vi "Initialize.vi"(0 "VISA resource name":refnum<visa-resource-name>, 1 "ID Query (True)":bool=TRUE, 2 "Reset (False)":bool, 3 "error in (no error)":errorcluster, 4 "Serial Link (RS232)":enum16{"RS232", "USB"}(ring)) -> (7 "VISA resource name out":refnum<visa-resource-name>, 8 "Cleared Error Queue":string, 10 "error out":errorcluster {"code" format="%.0x"})   [LabVIEW 2011, in "Newport ESP301.lvlib"]
doc: "Establishes communication with the instrument and optionally performs an instrument identification query and/or an instrument reset. It also places the instrument in a default state needed for other instrument driver operations. Therefore, call this VI before calling other instrument driver VIs for this instrument. Generally, you need to call the Initialize VI only once at the beginning of an application."
uses:
  Newport ESP301.lvlib
panel:
  # "(c) 2009 <Newport>.  ALL RIGHTS RESERVED."
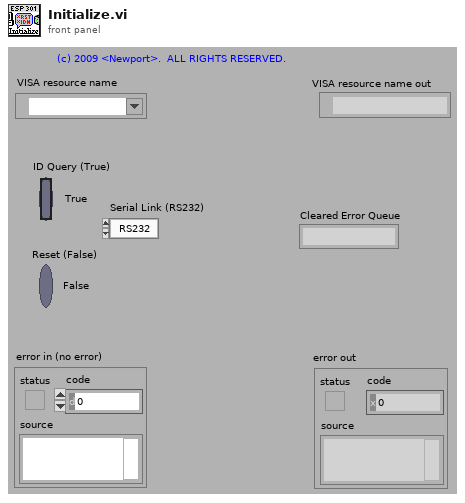
[diagram p1: front panel]
types:
  T1 = cluster{"Baud Rate":u32, "Parity":u16, "Data Bits":u16, "Stop Bits":u16, "Flow Control":u16}
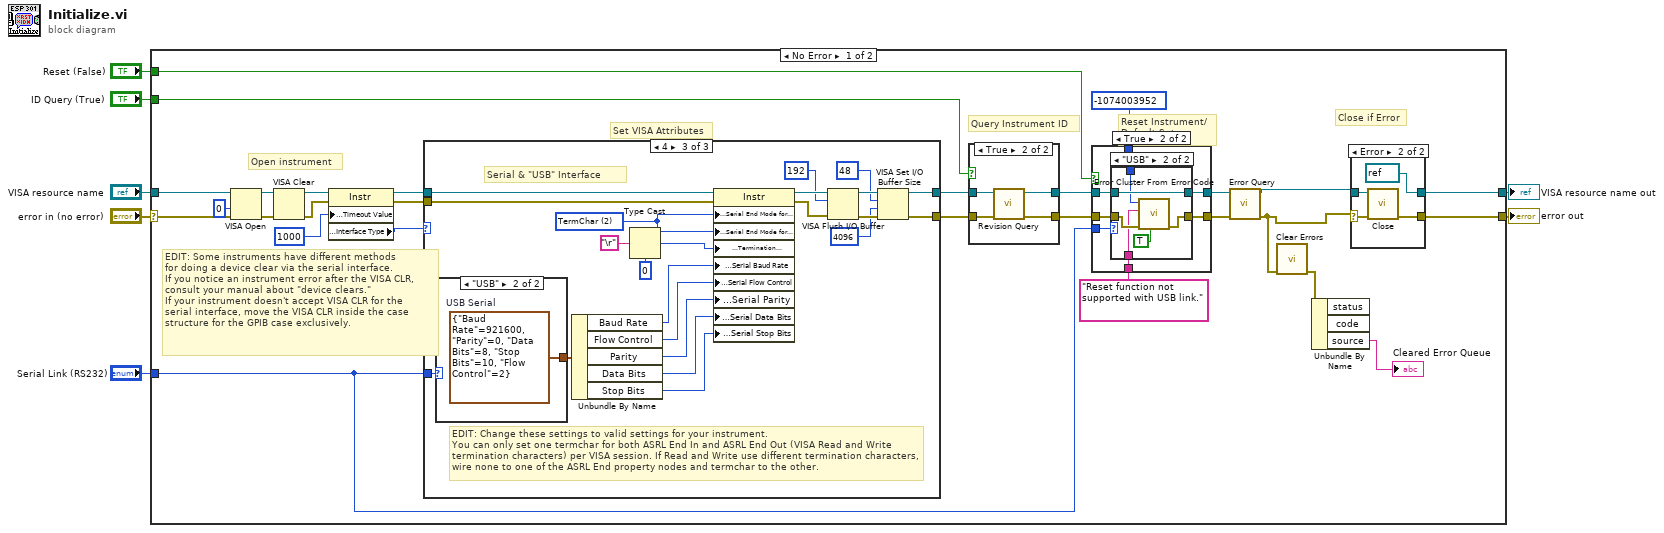
[diagram p0: block diagram]
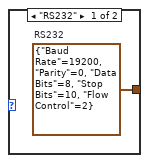
[diagram p5: hidden frame]
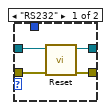
[diagram p7: hidden frame]
diagram:
  n1 = case shown="No Error" "error in (no error)" {
    selector: "error in (no error)" -> [w17 w96]
    tunnel: "ID Query (True)" -> [w33 _]
    tunnel: "Reset (False)" -> [w32 _]
    tunnel: "VISA resource name" -> [w31 w95]
    tunnel: [w15 w95] -> w4
    tunnel: [w16 w96] -> w3
    tunnel: "Serial Link (RS232)" -> [w14 _]
    frame No Error {
      # "EDIT: Some instruments have different methods\nfor doing a device clear via the serial interface.  \nIf you notice an instrument error after the VISA CLR,\nconsult your manual about \"device clears.\"  \nIf your instrument doesn't accept VISA CLR for the\nserial interface, move the VISA CLR inside the case \nstructure for the GPIB case exclusively."
      # "Set VISA Attributes"
      # "Close if Error"
      # "Query Instrument ID"
      # "Reset Instrument/\nDefault Setup"
      # "Open instrument"
      n2 = VISA Open(access mode=u32 0, error in (no error)=w17, VISA resource name=w31) -> (VISA resource name=w24:refnum<visa-resource-name>, error out=w23:errorcluster)  [unwired: 2 out]
      n3 = VISA Clear(VISA resource name=w24, error in (no error)=w23) -> (VISA resource name out=w22:refnum<visa-resource-name>, error out=w21:errorcluster)
      n4 = property class="Instr"(reference=w22, error in=w21, "General Settings:Timeout Value"=u32 1000) -> (reference out=w27:refnum<visa-resource-name>, error out=w26:errorcluster, "Interface Information:Interface Type"=w18:u16)
      n5 = case shown="4" w18 {
        tunnel: [w42 w45 w64] -> w29
        tunnel: [w43 w44 w61] -> w28
        tunnel: w27 -> [w42 w45 w66]
        tunnel: w26 -> [w43 w44 w67]
        tunnel: w14 -> [_ _ w48]
        frame Default {
          # "TCP/IP, and USB Interface"
        }
        frame 1 {
          # "GPIB Interface"
        }
        frame 4 {
          w55 = u16 2 items=["None", "LastBit", "TermChar"] ("Serial Settings:Serial End Mode for Reads")
          # "EDIT: Change these settings to valid settings for your instrument.\nYou can only set one termchar for both ASRL End In and ASRL End Out (VISA Read and Write termination characters) per VISA session. If Read and Write use different termination characters, wire none to one of the ASRL End property nodes and termchar to the other."
          # "Serial & \"USB\" Interface"
          n6 = case shown="\"USB\"" w48 {
            tunnel: [w68 w69] -> w47
            frame "RS232" {
              w68 = T1 {"Baud Rate"=19200, "Parity"=0, "Data Bits"=8, "Stop Bits"=10, "Flow Control"=2}  # RS232
            }
            frame "USB" {
              w69 = T1 {"Baud Rate"=921600, "Parity"=0, "Data Bits"=8, "Stop Bits"=10, "Flow Control"=2}  # USB Serial
            }
          }
          n7 = Unbundle By Name(w47) -> ("Baud Rate"=w53:u32, "Flow Control"=w50:u16, "Parity"=w51:u16, "Data Bits"=w52:u16, "Stop Bits"=w49:u16)
          n8 = Type Cast(type=u8 0, x="\r") -> (*(type *) &x=w54:u8)
          n9 = property class="Instr"(reference=w66, error in=w67, "Serial Settings:Serial End Mode for Reads"=w55, "Serial Settings:Serial End Mode for Writes"=w55, "Message Based Settings:Termination Character"=w54, "Serial Settings:Serial Baud Rate"=w53, "Serial Settings:Serial Flow Control"=w50, "Serial Settings:Serial Parity"=w51, "Serial Settings:Serial Data Bits"=w52, "Serial Settings:Serial Stop Bits"=w49) -> (reference out=w60:refnum<visa-resource-name>, error out=w63:errorcluster)
          n10 = VISA Flush I/O Buffer(VISA resource name=w60, mask (16)=u16 192, error in (no error)=w63) -> (VISA resource name out=w65:refnum<visa-resource-name>, error out=w62:errorcluster)
          n11 = VISA Set I/O Buffer Size(VISA resource name=w65, mask (16)=u16 48, size (4096)=u32 4096 ("size (0)"), error in (no error)=w62) -> (VISA resource name out=w64:refnum<visa-resource-name>, error out=w61:errorcluster)
        }
      }
      n12 = case shown="True" w33 {
        tunnel: [w89 w91] -> w34
        tunnel: [w90 w93] -> w35
        tunnel: w29 -> [w90 w94]
        tunnel: w28 -> [w89 w92]
        frame False {
        }
        frame True {
          n13 = call "Revision Query.vi"("error in (no error)"=w92, "VISA resource name"=w94) -> ("error out"=w91:errorcluster, "VISA resource name out"=w93:refnum<visa-resource-name>)  [unwired: 8 out]
        }
      }
      n14 = case shown="True" w32 {
        tunnel: w34 -> [w70 w75]
        tunnel: [w70 w78] -> w19
        tunnel: w35 -> [w71 w76]
        tunnel: [w71 w77] -> w20
        tunnel: w14 -> [_ w74]
        tunnel: -1074003952 ("Code") -> [_ w73]
        tunnel: "Reset function not supported with USB link." ("Source (VI Name)") -> [_ w72]
        frame False {
        }
        frame True {
          n15 = case shown="\"USB\"" w74 {
            tunnel: [w82 w85] -> w78
            tunnel: [w81 w88] -> w77
            tunnel: w76 -> [w80 w88]
            tunnel: w75 -> [w79 w86]
            tunnel: w73 -> [_ w84]
            tunnel: w72 -> [_ w83]
            frame "RS232" {
              n16 = call "Reset.vi"("error in (no error)"=w79, "VISA resource name"=w80) -> ("error out"=w82:errorcluster, "VISA resource name out"=w81:refnum<visa-resource-name>)  [unwired: 4 out]
            }
            frame "USB" {
              n17 = call "Error Cluster From Error Code.vi"("show call chain? (False)"=TRUE, "error in (no error)"=w86, "error message (\"\")"=w83, "error code (0)"=w84) -> ("error out"=w85:errorcluster)  [unwired: 5 out]
            }
          }
        }
      }
      n18 = call "Error Query.vi"("error in (no error)"=w19, "VISA resource name"=w20) -> ("error out"=w9:errorcluster, "VISA resource name out"=w8:refnum<visa-resource-name>)  [unwired: 4 out]
      n19 = call "Clear Errors.vi"("error in (no error)"=w9) -> ("error out"=w11:errorcluster)  [unwired: 6 in]
      n20 = Unbundle By Name(w11) -> ("source"=→"Cleared Error Queue":string)  [unwired: 2 out]
      n21 = case shown="Error" w9 {
        selector: w9 -> [w37 w39]
        tunnel: w8 -> [w36 w40]
        tunnel: [w36 refnum<visa-resource-name> refnum ("VISA resource name out")] -> w15
        tunnel: [w37 w41] -> w16
        frame No Error {
        }
        frame Error {
          n22 = call "Close.vi"("error in (no error)"=w39, "VISA resource name"=w40) -> ("error out"=w41:errorcluster)  [unwired: 9 out]
        }
      }
    }
    frame Error {
    }
  }
  "VISA resource name out" <- w4
  "error out" <- w3
